vi "Get Fonts Installed.vi"() -> (0 "error out":errorcluster, 3 "System Fonts [ ]":string[](array[string]))   [LabVIEW 2020]
uses:
  <vilib>/registry/registry.llb/Registry RtKey.ctl
  <vilib>/registry/registry.llb/Registry SAM.ctl
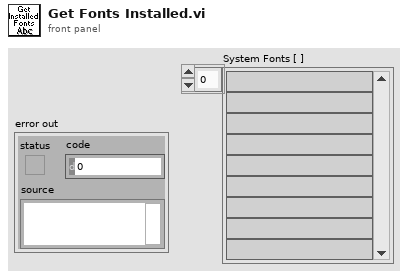
[diagram p1: front panel]
types:
  T1 = typedef "Registry SAM.ctl" = enum32{"KEY_QUERY_VALUE", "KEY_SET_VALUE", "KEY_CREATE_SUB_KEY", "KEY_ENUMERATE_SUB_KEYS", "KEY_NOTIFY", "KEY_CREATE_LINK", "KEY_READ", "KEY_WRITE", "KEY_ALL_ACCESS", "KEY_READ | KEY_WRITE"}
  T2 = typedef "Registry RtKey.ctl" = enum32{"HKEY_CLASSES_ROOT", "HKEY_CURRENT_USER", "HKEY_LOCAL_MACHINE", "HKEY_USERS", "HKEY_PERFORMANCE_DATA", "HKEY_CURRENT_CONFIG", "HKEY_DYN_DATA"}
  T3 = typedef "Registry refnum.ctl" = refnum<k1>
  T4 = cluster{"numValues":i32, "maxValueNameLen":i32, "maxValueDataLen":i32}
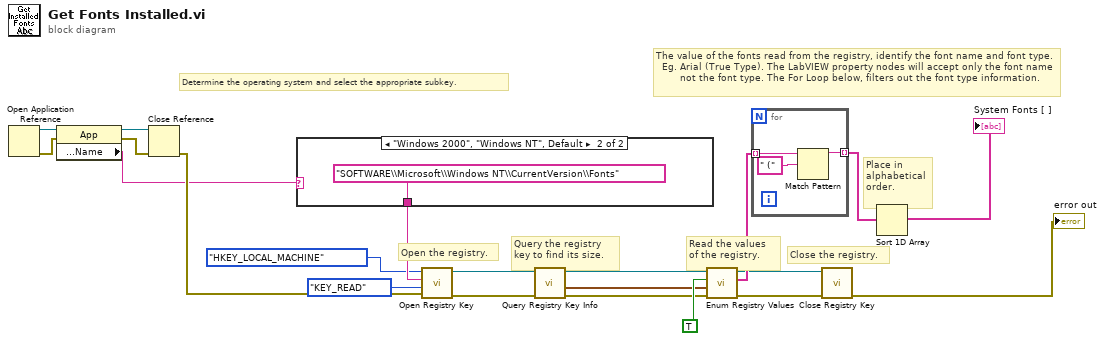
[diagram p0: block diagram]
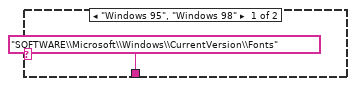
[diagram p2: hidden frame]
diagram:
  # "Determine the operating system and select the appropriate subkey."
  # "Place in \nalphabetical\norder."
  # "The value of the fonts read from the registry, identify the font name and font type. \n  Eg. Arial (True Type). The LabVIEW property nodes will accept only the font name\n        not the font type. The For Loop below, filters out the font type information."
  # "Close the registry."
  # "Query the registry \nkey to find its size."
  # "Open the registry."
  # "Read the values \nof the registry."
  n1 = Open Application Reference() -> (0:w16:errorcluster, 3:w15:refnum<vi>)  [unwired: 4 in]
  n2 = property class="App"(reference=w15, error in=w16) -> (reference out=w20:refnum<vi>, error out=w19:errorcluster, "Operating System:Name"=w17:string)
  n3 = Close Reference(reference=w20, error in (no error)=w19) -> (error out=w21:errorcluster)
  n4 = case shown="\"Windows 2000\", \"Windows NT\", Default" w17 {
    tunnel: ["SOFTWARE\\Microsoft\\Windows\\CurrentVersion\\Fonts" ("subkey") "SOFTWARE\\Microsoft\\Windows NT\\CurrentVersion\\Fonts" ("subkey")] -> w18
    frame "Windows 95", "Windows 98" {
    }
    frame "Windows 2000", "Windows NT", Default {
    }
  }
  n5 = call <vilib>:"Open Registry Key.vi"("error in (no error)"=w21, "security access mask (KEY_READ | KEY_WRITE)"=Registry_SAM."KEY_READ", "subkey"=w18, "root key (HKEY_LOCAL_MACHINE)"=Registry_RtKey."HKEY_LOCAL_MACHINE") -> ("error out"=w3:errorcluster, "refnum out"=w4:T3)  [unwired: 6 in]
  n6 = call <vilib>:"Query Registry Key Info.vi"("error in (no error)"=w3, "refnum"=w4) -> ("error out"=w7:errorcluster, "value info"=w6:T4, "refnum out"=w5:T3)  [unwired: 5 in, 2 out]
  n7 = call <vilib>:"Enum Registry Values.vi"("error in (no error)"=w7, "value info"=w6, "retrieve data? (F)"=TRUE, "refnum"=w5) -> ("error out"=w9:errorcluster, "values"=w12:string[], "refnum out"=w8:T3)  [unwired: 2 in, 3 out]
  n8 = for {
    tunnel: w12 -> [w26] mode=indexing
    tunnel: [w25] -> w13 mode=indexing
    n9 = Match Pattern(string=w26, regular expression=" (") -> (before substring=w25:string)  [unwired: 1 in, 3 out]
  }
  n10 = call <vilib>:"Close Registry Key.vi"("error in (no error)"=w9, "refnum"=w8) -> ("error out"=→"error out":errorcluster)  [unwired: 5 in]
  n11 = Sort 1D Array(array=w13) -> (sorted array=→"System Fonts [ ]":string[])
